vi "GetPowerMeasurement.vi"(7 "Frequency (Hz)":dbl=100000000.0 format="%#_6p", 8 "error in (no error)":errorcluster, 9 "Level (dBm)":dbl format="%#_13g", 10 "Alias":string="PwrSensor_1", 11 "PwrMtr_U2k.lvclass.In":refnum<class "PwrMtr_U2k.lvclass">) -> (0 "error out":errorcluster, 2 "Power (dBm)":dbl, 3 "PwrMtr_U2k.lvclass.Out":refnum<class "PwrMtr_U2k.lvclass">)   [LabVIEW 2014, in "PwrMtr_U2k.lvclass"]
uses:
  PwrMtr_U2k.lvclass
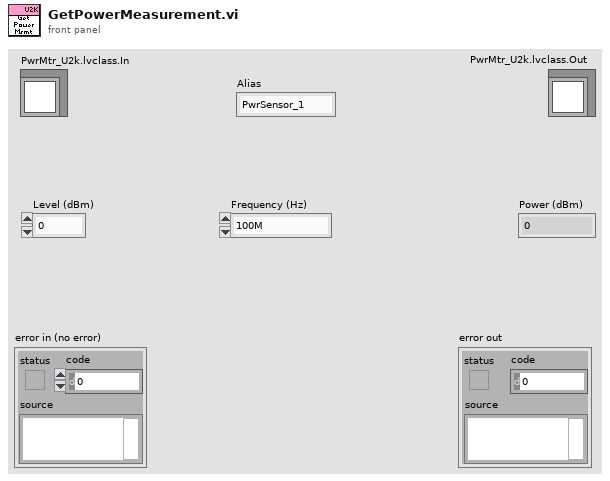
[diagram p1: front panel]
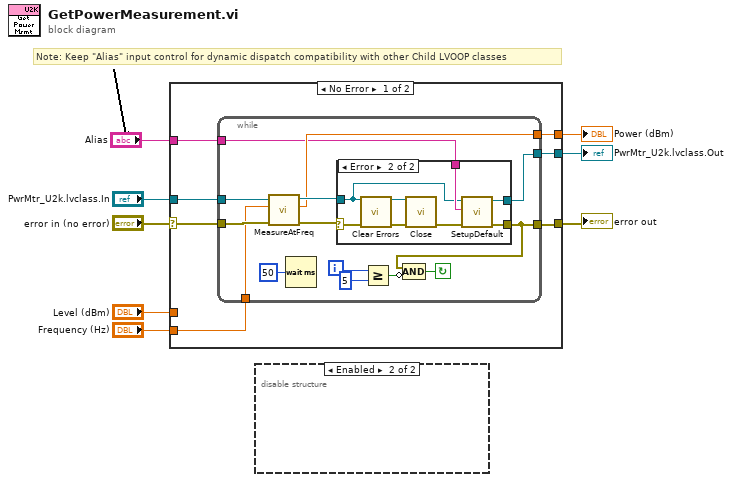
[diagram p0: block diagram]
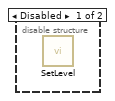
[diagram p2: hidden frame]
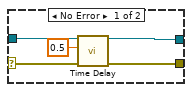
[diagram p3: hidden frame]
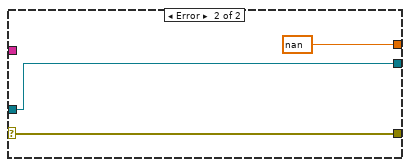
[diagram p4: hidden frame]
diagram:
  # "Note: Keep \"Alias\" input control for dynamic dispatch compatibility with other Child LVOOP classes"
  n1 = case shown="No Error" "error in (no error)" {
    selector: "error in (no error)" -> [w14 w43]
    tunnel: "Frequency (Hz)" -> [w11 _]
    tunnel: [w9 w42] -> w7
    tunnel: [w12 nan ("Power (dBm)")] -> w6
    tunnel: [w10 w43] -> w5
    tunnel: "Level (dBm)" -> [_ _]
    tunnel: "PwrMtr_U2k.lvclass.In" -> [w13 w42]
    tunnel: "Alias" -> [w15 _]
    frame No Error {
      n2 = while {
        tunnel: [w25] -> w10
        tunnel: w14 -> [w23]
        tunnel: w13 -> [w17]
        tunnel: w15 -> [w18]
        tunnel: [w16] -> w9
        tunnel: [w20] -> w12
        tunnel: w11 -> [w19]
        i -> [w28]
        stop <- w24 continue-if-true
        n3 = call-dynamic "MeasureAtFreq.vi"("error in (no error)"=w23, "Frequency (Hz)"=w19, "PwrMtr_U2k in"=w17) -> ("error out"=w22:errorcluster, "Power (dBm)"=w20:dbl, "PwrMtr_U2k out"=w21:refnum<class "PwrMtr_U2k.lvclass">)  [unwired: 6 in]
        n4 = Wait (ms)(milliseconds to wait=u32 50) -> ()  [unwired: 1 out]
        n5 = case shown="Error" w22 {
          selector: w22 -> [w33 w40]
          tunnel: [w32 w37] -> w25
          tunnel: w21 -> [w30 w35]
          tunnel: w18 -> [_ w36]
          tunnel: [w30 w34] -> w16
          frame No Error {
            n6 = call "Time Delay"("error in (no error)"=w33, "Delay Time (s)"=0.5) -> ("error out"=w32:errorcluster)  [unwired: 9 in]
          }
          frame Error {
            n7 = call <vilib>:"Clear Errors.vi"("error in (no error)"=w40) -> ("error out"=w39:errorcluster)  [unwired: 5 in, 1 out]
            n8 = call-dynamic "Close.vi"("error in (no error)"=w39, "PwrMtr_U2k in"=w35) -> ("error out"=w38:errorcluster)  [unwired: 9 in]
            n9 = call-dynamic "SetupDefault.vi"("error in (no error)"=w38, "Alias"=w36, "PwrMtr_U2k in"=w35) -> ("error out"=w37:errorcluster, "PwrMtr_U2k out"=w34:refnum<class "PwrMtr_U2k.lvclass">)  [unwired: 7 in]
          }
        }
        n10 = Greater Or Equal?(x=w28, y=5) -> (x >= y?=w26:bool)
        n11 = Compound Arithmetic op=AND(w25, invert w26) -> (w24:bool)
      }
    }
    frame Error {
    }
  }
  "PwrMtr_U2k.lvclass.Out" <- w7
  "Power (dBm)" <- w6
  "error out" <- w5
  n12 = disable-structure shown="Enabled" {
    frame Disabled {
      n13 = call-dynamic "SetLevel.vi"() -> ()  [unwired: 10 in, 2 out]
    }
    frame Enabled {
    }
  }
